vi "Read View Details.vi"(7 "error in (no error)":errorcluster, 9 "View Name":string, 10 "Controller Actor in":refnum<class "Controller Actor.lvclass">) -> (0 "error out":errorcluster, 1 "View Not Found":bool, 2 "View Details":T1, 3 "Controller Actor out":refnum<class "Controller Actor.lvclass">)   [LabVIEW 2017, in "Event Actors.lvlib" / "Controller Actor.lvclass"]
doc: "Allows the child controller to get the behavior of a View actor specified in the <b>View Name</b> by registering to the user defined event whose reference is accessible by the <b>View Settings Event Ref</b> property that will deliver the following settings:\n\n<b>Exclude From Broadcast</b>: message originating form another sink will not be broadcasted to the sink being cosidered\n<b>Paused</b>: the sink will not send events and will not receive them anymore\n<b>Receive only</b>: The sing will receive events but not send any"
uses:
  Controller Actor.lvclass
  View Details.ctl
  <vilib>/ActorFramework/Message Enqueuer/Message Enqueuer.lvclass
  Controller Actor.lvclass/Controller Actor.ctl
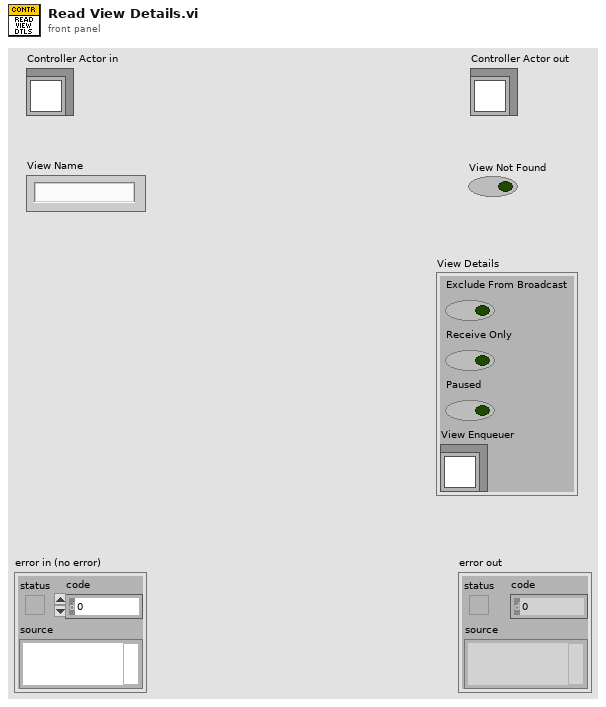
[diagram p1: front panel]
types:
  T1 = typedef "Event Actors.lvlib/Controller Actor.lvclass/View Details.ctl" = cluster{"Exclude From Broadcast":bool, "Receive Only":bool, "Paused":bool, "View Enqueuer":refnum<class "Message Enqueuer.lvclass">}
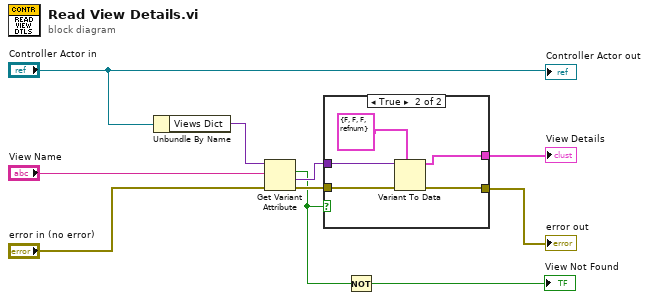
[diagram p0: block diagram]
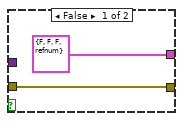
[diagram p2: hidden frame]
diagram:
  n1 = Unbundle By Name("Controller Actor in") -> ("Views Dict"=w8:variant)
  n2 = Get Variant Attribute(Variant=w8, name="View Name", error in="error in (no error)") -> (found=w3:bool, value=w9:variant, error out=w10:errorcluster)  [unwired: 1 in, 1 out]
  n3 = case shown="True" w3 {
    tunnel: w9 -> [_ w16]
    tunnel: w10 -> [w12 w17]
    tunnel: [w12 w14] -> w4
    tunnel: [T1 {"Exclude From Broadcast"=FALSE, "Receive Only"=FALSE, "Paused"=FALSE, "View Enqueuer"=refnum} ("Message Enqueuer") w13] -> w1
    frame False {
    }
    frame True {
      n4 = Variant To Data(error in=w17, type=T1 {"Exclude From Broadcast"=FALSE, "Receive Only"=FALSE, "Paused"=FALSE, "View Enqueuer"=refnum} ("Message Enqueuer"), Variant=w16) -> (data=w13:T1, error out=w14:errorcluster)
    }
  }
  "error out" <- w4
  "View Details" <- w1
  n5 = Not(x=w3) -> (.not. x?=→"View Not Found":bool)
  "Controller Actor out" <- "Controller Actor in"
